vi "Puertas_Abiertas_3gdl.vi"() -> ()   [LabVIEW 2014]
uses:
  <vilib>/Platform/TimedLoop/XDataNode/timing_clust.ctl
  <vilib>/Platform/TimedLoop/XDataNode/nitl_modes.ctl
  <vilib>/Platform/TimedLoop/XDataNode/wakeup.ctl
  <vilib>/Analysis/baseanly.llb/Real A x B.vi
  <vilib>/Platform/TimedLoop/XDataNode/loadnilvce.vi
  <vilib>/Analysis/Matrix/Numeric/Conversions/Array To Matrix - RA2.vi
  <vilib>/Analysis/Matrix/Numeric/Conversions/Array To Matrix - RA.vi
  <vilib>/Motion/Express/_s/nimc.ex.read.readExecutionData.axis.vi
  Global_Inicial.vi
  <vilib>/platform/TimedLoop/XDataNode/XDataNode.xnode
  <vilib>/Motion/BlockNode/FB.NIMotion.xnode
  <vilib>/Platform/TimedLoop/XDataNode/XDNodeRunTimeDep.lvlib
  <vilib>/ptbypt/NI_PtbyPt.lvlib
  <vilib>/Analysis/NI_AALBase.lvlib
  <vilib>/Analysis/Matrix/NI_Matrix.lvlib
panel:
  in  "stop 2":bool
  in  "stop":bool
  out "pkt":bool
  out "Posición FEH":dbl
  out "Posición RotIEH":dbl
  out "Posición FEC":dbl
  out "error out":errorcluster
  out "position °":dbl
  out "inicial":dbl format="%#_13g"
  out "Pos ant":dbl
  out "V MOTOR abajo":dbl
  out "Pos ant 1":dbl
  out "qd - sin":dbl
  out "tau 1":dbl
  out "Time":u32
  out "Motor abajo":dynamicdata(graph)
  in  "Kp":dbl=40.0
  in  "M_p":dbl=14.0
  in  "Kd":dbl=40.0
  out "Error imp 1":dbl[](graph)
  out "inicial 2":dbl format="%#_13g"
  out "Pos ant 2":dbl
  out "position ° 2":dbl
  out "Pos ant 2_2":dbl
  out "Motor medio":dynamicdata(graph)
  out "Error imp 2":dbl[](graph)
  out "Motor superior":dynamicdata(graph)
  out "inicial 3":dbl format="%#_13g"
  out "Pos ant 3":dbl
  out "position ° 3":dbl
  out "Pos ant 3_3":dbl
  out "q1":dbl
  out "qhp1":dbl
  out "qhpp1":dbl
  out "qhpp2":dbl
  out "qhp2":dbl
  out "q2":dbl
  out "qhpp3":dbl
  out "qhp3":dbl
  out "q3":dbl
  out "V MOTOR medio":dbl
  out "tau 2":dbl
  out "V MOTOR  superior":dbl
  out "tau 3":dbl
  out "Trayectoria qd 1":dbl[](array[numeric])
  out "Trayectoria qd 2":dbl[](array[numeric])
  out "Trayectoria qd 3":dbl[](array[numeric])
  out "qe cal 2":dbl
  out "Error imp 3":dbl[](graph)
  in  "epsilon 2":dbl=0.001 format="%#_13g"
  in  "epsilon 1":dbl=0.001 format="%#_13g"
  in  "epsilon 3":dbl=0.01 format="%#_13g"
  in  "sat 1":dbl=2.0
  in  "sat 2":dbl=2.0
  in  "sat 3":dbl=2.0
  in  "sat 4":dbl=2.0
  in  "sat 5":dbl=2.0
  in  "sat 6":dbl=0.0001
  in  "sat 7":dbl=0.0001
  in  "sat 8":dbl=2.0
  in  "sat 9":dbl=2.0
  in  "sat 10":dbl=2.0
  in  "sat 11":dbl=2.0
  in  "sat 12":dbl=2.0
  in  "sat 13":dbl=2.0
  in  "sat 14":dbl=2.0
  in  "sat 15":dbl=2.0
  in  "sat 16":dbl=2.0
  in  "sat 17":dbl=0.001
  in  "sat 18":dbl=5.0
  in  "sat 19":dbl=2.0
  in  "sat 20":dbl=2.0
  in  "sat 21":dbl=2.0
  in  "g 1":dbl=10.0
  in  "g 2":dbl=10.0
  in  "g 3":dbl=10.0
  in  "g 4":dbl=10.0
  in  "g 5":dbl=10.0
  in  "g 6":dbl=0.01
  in  "g 7":dbl=0.01
  in  "g 8":dbl=10.0
  in  "g 9":dbl=10.0
  in  "g 10":dbl=10.0
  in  "g 11":dbl=10.0
  in  "g 12":dbl=10.0
  in  "g 13":dbl=10.0
  in  "g 14":dbl=10.0
  in  "g 15":dbl=10.0
  in  "g 16":dbl=10.0
  in  "g 17":dbl=10.0
  in  "g 18":dbl=10.0
  in  "g 19":dbl=10.0
  in  "g 20":dbl=10.0
  in  "g 21":dbl=10.0
  out "i":i32
  out "Y":dbl[][](array[numeric])
  out "Sp_kpE":dbl
  out "Sp_kpE 2":dbl
  out "Sp_kpE 3":dbl
  out "qe cal 1":dbl
  out "qe cal 3":dbl
  out "qd - sin 2":dbl
  in  "Kp 2":dbl=250.0
  in  "M_p 2":dbl=90.0
  in  "Kd 2":dbl=250.0
  out "qd - sin 3":dbl
  in  "Kp 3":dbl=100.0
  in  "M_p 3":dbl=20.0
  in  "Kd 3":dbl=100.0
  in  "timeout ms (25000)":i32=100
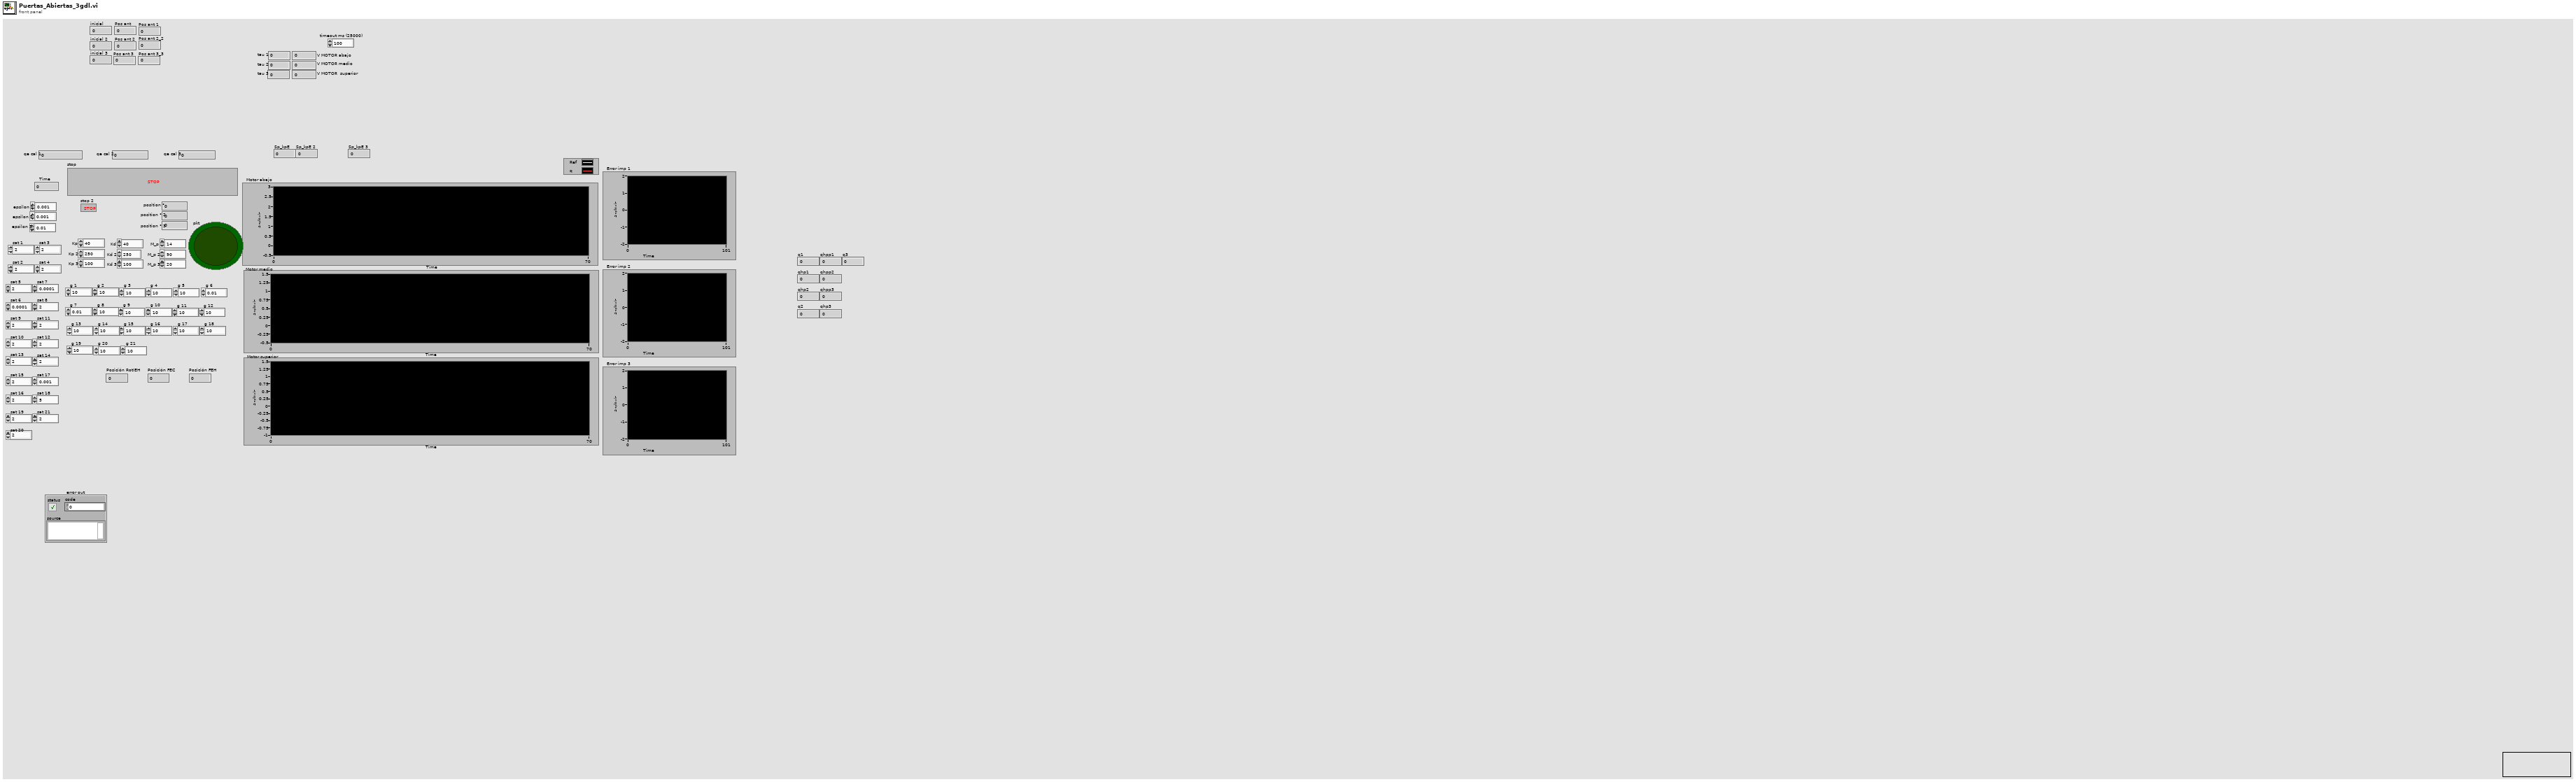
[diagram p1: front panel]
types:
  T1 = typedef "XDNodeRunTimeDep.lvlib/timing_clust.ctl" = cluster{"Expected End [f-1]":u64, "Actual End [f-1]":u64, "Finished Late? [f-1]":bool, "Expected End [i-1]":u64, "Actual End [i-1]":u64, "Finished Late? [i-1]":bool, "Expected Start [i]":u64, "Actual Start [i]":u64, "Expected Start [f]":u64, "Actual Start [f]":u64, "Source Name":string, "Structure Name":string, "Period":i64, "Deadline":i64, "Offset":i64, "Start":i64, "Priority":i32, "Timeout":i32, "Mode":T2, "Wakeup Reason":T3, "Error":errorcluster, "Source Type":string, "Secondary Source Type":string, "Global End Time":u64, "Global Start Time":u64, "Frame Duration":u64, "Iteration Duration":u64, "Assigned CPU":i32, "I/O Scan Engine Mode":u32}
  T2 = typedef "XDNodeRunTimeDep.lvlib/nitl_modes.ctl" = enum32{"No Change", "Process missed periods, maintain original phase", "Discard missed periods, maintain original phase", "Process missed periods, ignore original phase", "Discard missed periods, ignore original phase"}
  T3 = typedef "XDNodeRunTimeDep.lvlib/wakeup.ctl" = enum32{"Normal", "Aborted", "Asynchronous wakeup", "Timing source error", "Timed loop error", "Timeout"}
  T4 = typedef "NI_Matrix.lvlib/RealMatrix.ctl" = dbl[][]
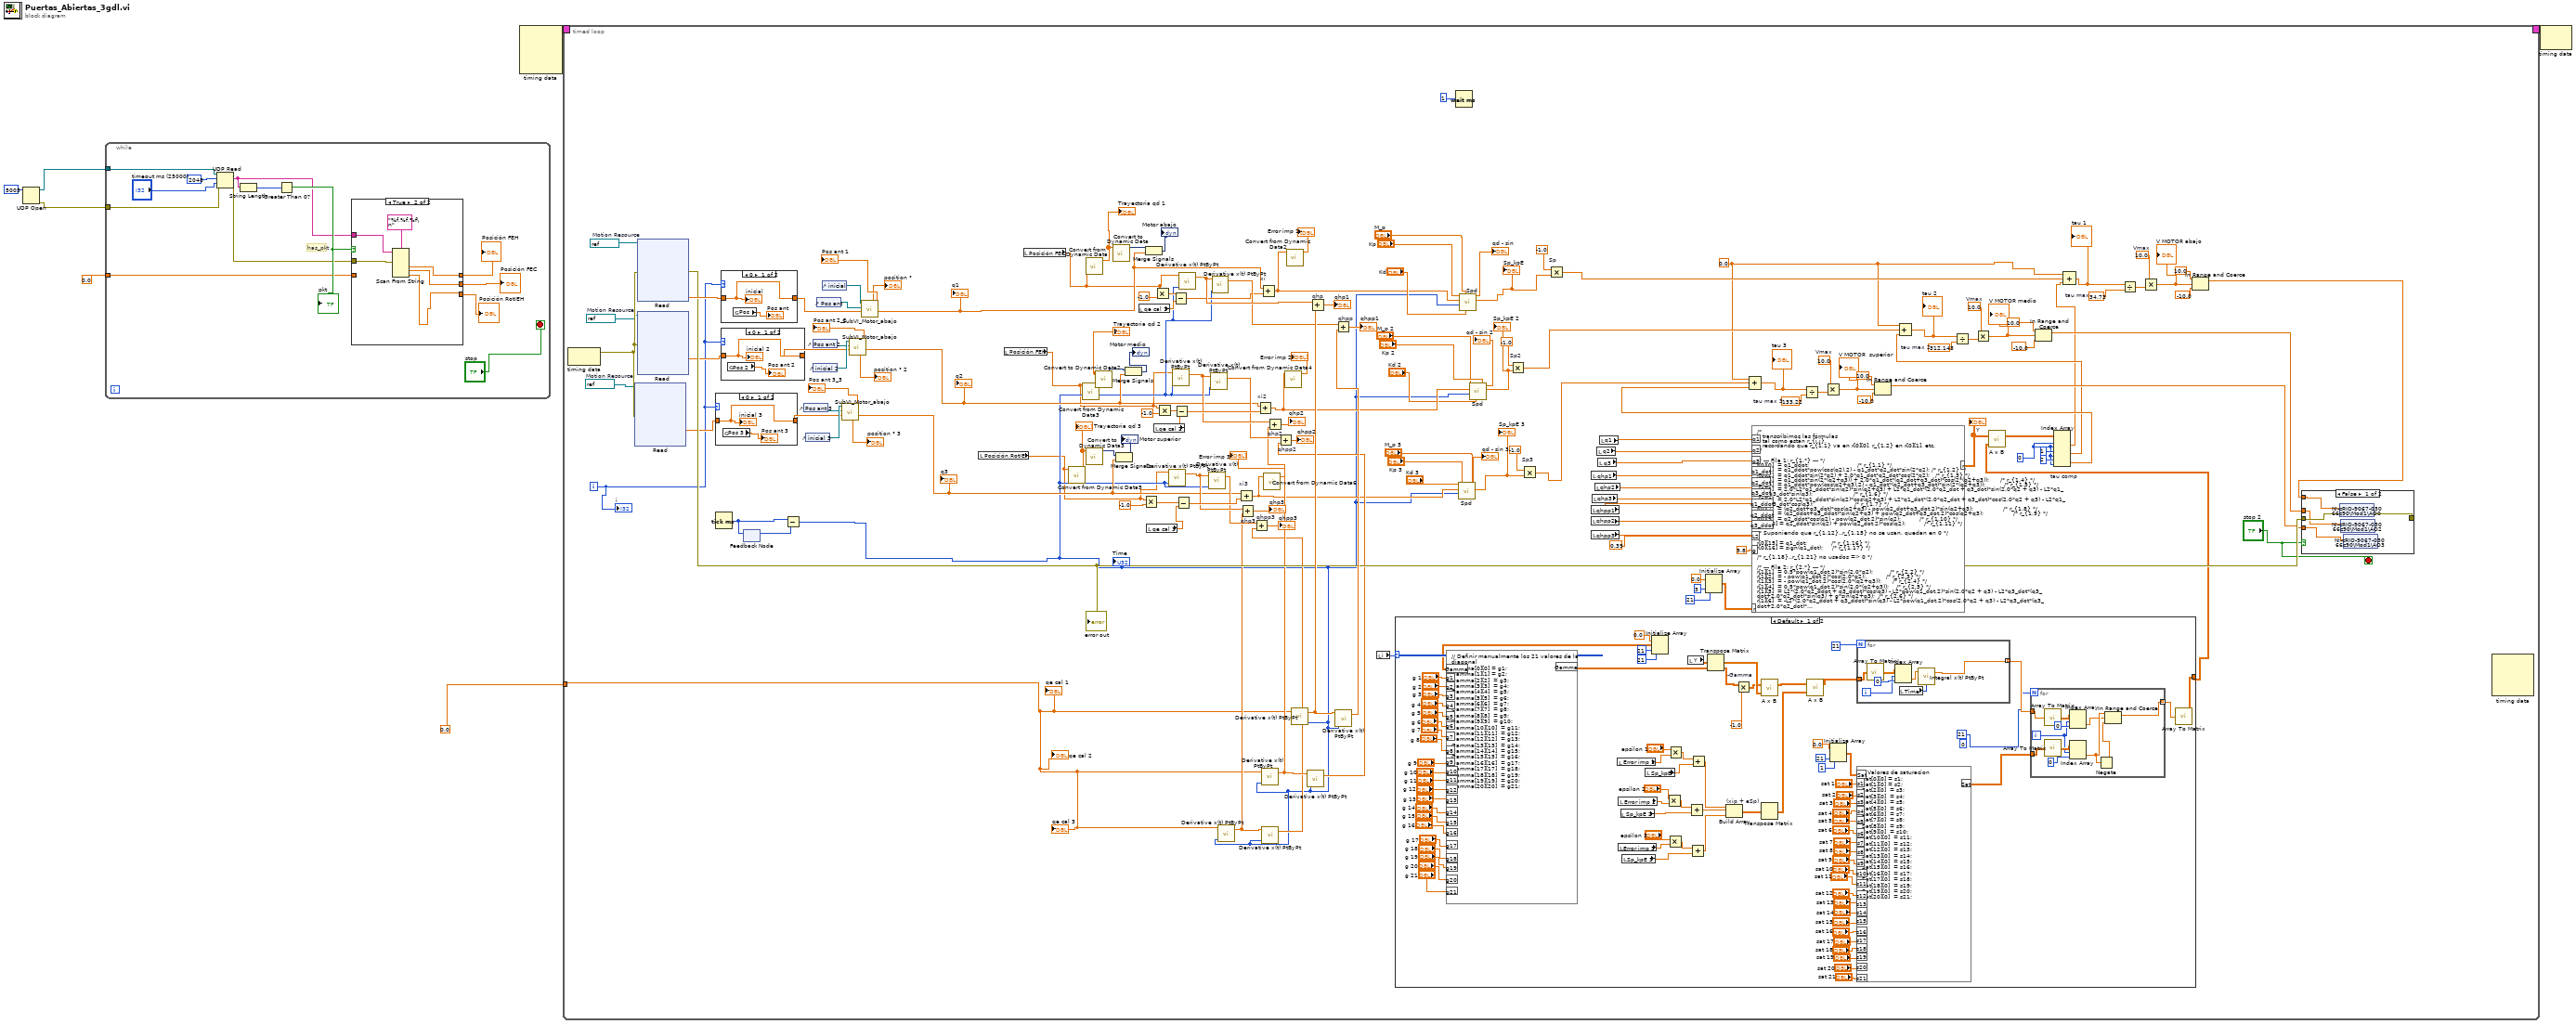
[diagram p0: block diagram]
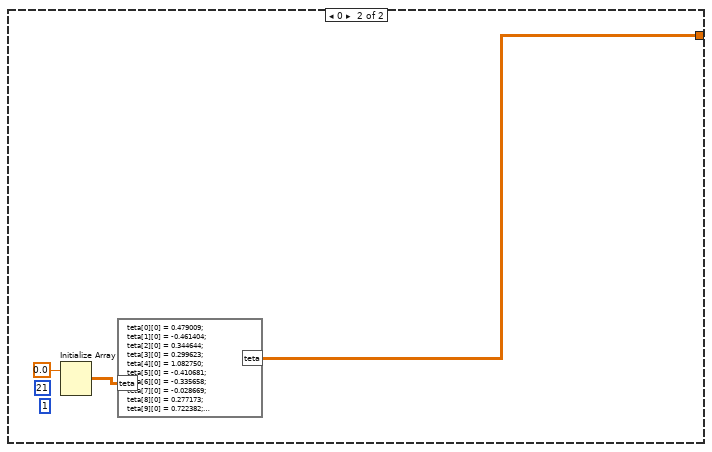
[diagram p2: hidden frame]
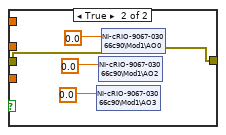
[diagram p5: hidden frame]
diagram:
  n1 = UDP Open(11:u16 5005 ("port")) -> (port=w6:refnum<k16>, 0:w7:errorcluster)  [unwired: 4 in, 1 out]
  n2 = while {
    tunnel: w7 -> [w17]
    tunnel: w6 -> [w16]
    tunnel: 0.0 -> [w11]
    stop <- "stop" stop-if-true
    # "has_pkt"
    n3 = UDP Read(connection ID=w16, max size (548)=2048, timeout ms (25000)="timeout ms (25000)", 8:w17) -> (data out=w13:string, error out=w12:errorcluster)  [unwired: 3 out]
    n4 = String Length(string=w13) -> (length=w18:i32)
    n5 = Greater Than 0?(x=w18) -> (x > 0?=w14:bool)
    "pkt" <- w14
    n6 = case shown="True" w14 {
      tunnel: w12 -> [_ w27]
      tunnel: w13 -> [_ w26]
      tunnel: [w21 w24] -> w15
      tunnel: w11 -> [w21 _]
      tunnel: [w21 w23] -> w10
      tunnel: [w21 w22] -> w9
      frame False {
      }
      frame True {
        n7 = Scan From String "Scan From String"(format string="%f,%f,%f\n", input string=w26, error in=w27) -> (output 1=w24:dbl, output 2=w23:dbl, output 3=w22:dbl)  [unwired: 4 in, 3 out]
      }
    }
    "Posición FEC" <- w10
    "Posición RotIEH" <- w9
    "Posición FEH" <- w15
  }
  n8 = node-c288() -> (w3:T1)  [unwired: 4 in]
  n9 = timed-loop {
    timing: w3 -> [_]
    timing-out: [_] -> w2
    tunnel: 0.0 -> [w33]
    i -> [w67]
    stop <- "stop 2" stop-if-true
    w32 = 0.0
    w70 = refnum<k21> "Axis 3"  # Motion Resource
    w71 = refnum<k21> "Axis 2"  # Motion Resource
    w88 = 0 ("index (col)")
    w95 = 10.0  # Vmax
    w97 = 133.22  # tau max 3
    w102 = 10.0  # Vmax
    w104 = 312.143  # tau max 2
    w177 = 10.0  # Vmax
    w179 = 34.73  # tau max
    w157 = refnum<k21> "Axis 1"  # Motion Resource
    n10 = node-c288() -> (w152:errorcluster)  [unwired: 1 in]
    n11 = xnode ("Read")("resource"=w71, "error in"=w152) -> ("position"=w121:dbl)  [unwired: 6 out]
    n12 = xnode ("Read")("resource"=w157, "error in"=w152) -> ("position"=w176:dbl, "error out"=w166:errorcluster)  [unwired: 5 out]
    "error out" <- w166
    n13 = xnode ("Read")("resource"=w70, "error in"=w152) -> ("position"=w151:dbl)  [unwired: 6 out]
    n14 = case shown="0" w67 {
      tunnel: w121 -> [w282 w283]
      tunnel: [w282 w283] -> w122
      frame 0 {
        n15 = global read "Global_Inicial.vi" "Pos 3"() -> (→"Pos ant 3":dbl)
        "inicial 3" <- w282
      }
      frame Default {
      }
    }
    n16 = Tick Count (ms)() -> (millisecond timer value=w68:u32)
    n17 = case shown="0" w67 {
      tunnel: w176 -> [w316 w317]
      tunnel: [w316 w317] -> w175
      frame 0 {
        n18 = global read "Global_Inicial.vi" "Pos"() -> (→"Pos ant":dbl)
        "inicial" <- w316
      }
      frame Default {
      }
    }
    n19 = case shown="0" w67 {
      tunnel: w151 -> [w285 w286]
      tunnel: [w285 w286] -> w146
      frame 0 {
        n20 = global read "Global_Inicial.vi" "Pos 2"() -> (→"Pos ant 2":dbl)
        "inicial 2" <- w285
      }
      frame Default {
      }
    }
    n21 = feedback #1() -> (w69:u32)  [unwired: 1 in]
    n22 = feedback-in #1(w68) -> ()
    n23 = Subtract(x=w68, y=w69) -> (x-y=w37:u32)
    "Time" <- w37
    n24 = control-ref of="Pos ant 3"() -> (w125:refnum<vi>)
    n25 = control-ref of="inicial 3"() -> (w126:refnum<vi>)
    n26 = control-ref of="Pos ant 2"() -> (w149:refnum<vi>)
    n27 = control-ref of="inicial 2"() -> (w150:refnum<vi>)
    n28 = control-ref of="Pos ant"() -> (w155:refnum<vi>)
    n29 = control-ref of="inicial"() -> (w156:refnum<vi>)
    n30 = call "SubVI_Motor_abajo.vi"("position"=w122, "reference in"=w125, "Digital in"=w126) -> ("Numeric"=w77:dbl, "Pos ant 2"=→"Pos ant 3_3":dbl, "position °"=→"position ° 3":dbl)  [unwired: 5 in, 1 out]
    "q3" <- w77
    n31 = call "SubVI_Motor_abajo.vi"("position"=w146, "reference in"=w149, "Digital in"=w150) -> ("Numeric"=w59:dbl, "Pos ant 2"=→"Pos ant 2_2":dbl, "position °"=→"position ° 2":dbl)  [unwired: 5 in, 1 out]
    "q2" <- w59
    n32 = call "SubVI_Motor_abajo.vi"("position"=w175, "reference in"=w155, "Digital in"=w156) -> ("Numeric"=w140:dbl, "Pos ant 2"=→"Pos ant 1":dbl, "position °"=→"position °":dbl)  [unwired: 5 in, 1 out]
    "q1" <- w140
    n33 = local read "Posición RotIEH"() -> (w29:dbl)
    n34 = local read "Posición FEH"() -> (w31:dbl)
    n35 = local read "Posición FEC"() -> (w30:dbl)
    n36 = call "Convert from Dynamic Data5"("Dynamic Data Type"=w29) -> ("Array"=w79:dbl[])  [unwired: 3 in]
    "Trayectoria qd 3" <- w79
    n37 = call "Convert from Dynamic Data3"("Dynamic Data Type"=w31) -> ("Array"=w80:dbl[])  [unwired: 3 in]
    "Trayectoria qd 2" <- w80
    n38 = call "Convert from Dynamic Data"("Dynamic Data Type"=w30) -> ("Array"=w145:dbl[])  [unwired: 3 in]
    "Trayectoria qd 1" <- w145
    n39 = call "Convert to Dynamic Data3"("Array"=w79) -> ("Dynamic Data Type"=w135:dynamicdata)  [unwired: 3 in]
    n40 = call "Convert to Dynamic Data2"("Array"=w80) -> ("Dynamic Data Type"=w78:dynamicdata)  [unwired: 3 in]
    n41 = call "Convert to Dynamic Data"("Array"=w145) -> ("Dynamic Data Type"=w164:dynamicdata)  [unwired: 3 in]
    n42 = Merge Signals(w135, w77) -> (→"Motor superior":dynamicdata)
    n43 = Merge Signals(w78, w59) -> (→"Motor medio":dynamicdata)
    n44 = local read "qe cal 1"() -> (w58:dbl)
    n45 = Multiply(x=w29, y=-1.0) -> (x*y=w132:dbl)
    n46 = Merge Signals(w164, w140) -> (→"Motor abajo":dynamicdata)
    n47 = local read "qe cal 3"() -> (w56:dbl)
    n48 = local read "qe cal 2"() -> (w57:dbl)
    n49 = Multiply(x=w30, y=-1.0) -> (x*y=w162:dbl)
    n50 = Multiply(x=w31, y=-1.0) -> (x*y=w143:dbl)
    n51 = call <vilib>:"Derivative x(t) PtByPt.vi"("dt"=w37, "x"=w29) -> ("dx/dt"=w130:dbl)  [unwired: 2 in, 1 out]
    n52 = Subtract(x=w162, y=w58) -> (x-y=w161:dbl)
    n53 = call <vilib>:"Derivative x(t) PtByPt.vi"("dt"=w37, "x"=w31) -> ("dx/dt"=w138:dbl)  [unwired: 2 in, 1 out]
    n54 = Subtract(x=w143, y=w57) -> (x-y=w141:dbl)
    n55 = Subtract(x=w132, y=w56) -> (x-y=w131:dbl)
    n56 = call <vilib>:"Derivative x(t) PtByPt.vi"("dt"=w37, "x"=w30) -> ("dx/dt"=w170:dbl)  [unwired: 2 in, 1 out]
    n57 = call <vilib>:"Derivative x(t) PtByPt.vi"("dt"=w37, "x"=w130) -> ("dx/dt"=w129:dbl)  [unwired: 2 in, 1 out]
    n58 = call <vilib>:"Derivative x(t) PtByPt.vi"("dt"=w37, "x"=w138) -> ("dx/dt"=w137:dbl)  [unwired: 2 in, 1 out]
    n59 = call <vilib>:"Derivative x(t) PtByPt.vi"("dt"=w37, "x"=w170) -> ("dx/dt"=w168:dbl)  [unwired: 2 in, 1 out]
    n60 = call <vilib>:"Derivative x(t) PtByPt.vi"("dt"=w37, "x"=w33) -> ("dx/dt"=w82:dbl)  [unwired: 2 in, 1 out]
    n61 = Add "xi3"(x=w77, y=w131) -> (x+y=w38:dbl)
    n62 = Add "qhp3"(x=w130, y=w82) -> (x+y=→"qhp3":dbl)
    n63 = Add "xi2"(x=w59, y=w141) -> (x+y=w45:dbl)
    n64 = Add "xi"(x=w140, y=w161) -> (x+y=w51:dbl)
    n65 = call <vilib>:"Derivative x(t) PtByPt.vi"("dt"=w37, "x"=w33) -> ("dx/dt"=w84:dbl)  [unwired: 2 in, 1 out]
    n66 = call <vilib>:"Derivative x(t) PtByPt.vi"("dt"=w37, "x"=w82) -> ("dx/dt"=w81:dbl)  [unwired: 2 in, 1 out]
    n67 = Add "qhpp3"(x=w129, y=w81) -> (x+y=→"qhpp3":dbl)
    n68 = call "Convert from Dynamic Data6"("Dynamic Data Type"=w38) -> ("Array"=→"Error imp 3":dbl[])  [unwired: 3 in]
    n69 = Add "qhp2"(x=w138, y=w84) -> (x+y=→"qhp2":dbl)
    n70 = call "Convert from Dynamic Data4"("Dynamic Data Type"=w45) -> ("Array"=→"Error imp 2":dbl[])  [unwired: 3 in]
    n71 = call "Convert from Dynamic Data2"("Dynamic Data Type"=w51) -> ("Array"=→"Error imp 1":dbl[])  [unwired: 3 in]
    n72 = call <vilib>:"Derivative x(t) PtByPt.vi"("dt"=w37, "x"=w33) -> ("dx/dt"=w169:dbl)  [unwired: 2 in, 1 out]
    n73 = call <vilib>:"Derivative x(t) PtByPt.vi"("dt"=w37, "x"=w84) -> ("dx/dt"=w83:dbl)  [unwired: 2 in, 1 out]
    n74 = Add "qhpp2"(x=w137, y=w83) -> (x+y=→"qhpp2":dbl)
    n75 = Add "qhp"(x=w170, y=w169) -> (x+y=→"qhp1":dbl)
    n76 = call <vilib>:"Derivative x(t) PtByPt.vi"("dt"=w37, "x"=w169) -> ("dx/dt"=w167:dbl)  [unwired: 2 in, 1 out]
    n77 = Add "qhpp"(x=w168, y=w167) -> (x+y=→"qhpp1":dbl)
    n78 = local read "i"() -> (w66:i32)
    n79 = case shown="Default" w66 {
      tunnel: [w224 w278] -> w60
      frame Default {
        (unwired) 0 ("dimension size")
        n80 = local read "Error imp 1"() -> (w249:dbl[])
        n81 = local read "Error imp 3"() -> (w240:dbl[])
        n82 = local read "Error imp 2"() -> (w244:dbl[])
        n83 = local read "Sp_kpE 2"() -> (w243:dbl)
        n84 = local read "Sp_kpE 3"() -> (w239:dbl)
        n85 = local read "Sp_kpE"() -> (w247:dbl)
        n86 = Initialize Array(0.0 ("element"), 21 ("dimension size"), 21 ("dimension size")) -> (w255:dbl[][])
        n87 = formula code="// Definir manualmente los 21 valores de la diagonal\nGamma[0][0] = g1;\nGamma[1][1] = g2;\nGamma[2][2]  = g3;\nGamma[3][3]  = g4;\nGamma[4][4]  = g5;\nGamma[5][5]  = g6;\nGamma[6][6]  = g7;\nGamma[7][7]  = g8;\nGamma[8][8]  = g9;\nGamma[9][9]  = g10;\nGamma[10][10]  = g11;\nGamma[11][11]  = g12;\nGamma[12][12]  = g13;\nGamma[13][13]  = g14;\nGamma[14][14]  = g15;\nGamma[15][15]  = g16;\nGamma[16][16]  = g17;\nGamma[17][17]  = g18;\nGamma[18][18]  = g19;\nGamma[19][19]  = g20;\nGamma[20][20]  = g21;"("Gamma"=w255, "g1"="g 1", "g2"="g 2", "g3"="g 3", "g4"="g 4", "g5"="g 5", "g6"="g 6", "g7"="g 7", "g8"="g 8", "g9"="g 9", "g10"="g 10", "g11"="g 11", "g12"="g 12", "g13"="g 13", "g14"="g 14", "g15"="g 15", "g16"="g 16", "g17"="g 17", "g18"="g 18", "g19"="g 19", "g20"="g 20", "g21"="g 21") -> ("Gamma"=w253:dbl[][])
        n88 = Multiply(x="epsilon 2", y=w244) -> (x*y=w246:dbl[])
        n89 = Multiply(x="epsilon 3", y=w240) -> (x*y=w242:dbl[])
        n90 = Multiply(x="epsilon 1", y=w249) -> (x*y=w248:dbl[])
        n91 = local read "Y"() -> (w259:dbl[][])
        n92 = Add(x=w246, y=w243) -> (x+y=w237:dbl[])
        n93 = Add(x=w242, y=w239) -> (x+y=w236:dbl[])
        n94 = Add(x=w248, y=w247) -> (x+y=w238:dbl[])
        n95 = Transpose Matrix(1:w259) -> (0:w254:dbl[][])
        n96 = Build Array "(xip + eSp)"(w238, w237, w236) -> (w228:T4)
        n97 = Multiply "-Gamma"(x=w253, y=-1.0) -> (x*y=w252:dbl[][])
        n98 = Transpose Matrix(1:w228) -> (0:w227:T4)
        n99 = call-poly <vilib>:"A x B.vi"("B"=w254, "A"=w252) -> ("A x B"=w251:T4)  [unwired: 1 out]
        n100 = call-poly <vilib>:"A x B.vi"("B"=w227, "A"=w251) -> ("A x B"=w235:T4)  [unwired: 1 out]
        n101 = Initialize Array(0.0 ("element"), 21 ("dimension size"), 1 ("dimension size")) -> (w231:dbl[][])
        n102 = for {
          N: 21 ("dimension size") -> [_]
          tunnel: w235 -> [w273]
          tunnel: [w271] -> w226 mode=indexing
          i -> [w275]
          n103 = call-poly <vilib>:"Array To Matrix.vi"("Real 2D Array"=w273) -> ("Real Matrix"=w274:T4)
          n104 = Index Array(array=w274, index (row)=w275, index (col)=0) -> (element=w272:dbl)
          n105 = local read "Time"() -> (w276:u32)
          n106 = call <vilib>:"Integral x(t) PtByPt.vi"("dt"=w276, "x"=w272) -> ("integral x(t)"=w271:dbl)  [unwired: 2 in, 1 out]
        }
        n107 = formula code="// Valores de saturacion\nSat[0][0] = s1;\nSat[1][0] = s2;\nSat[2][0]  = s3;\nSat[3][0]  = s4;\nSat[4][0]  = s5;\nSat[5][0]  = s6;\nSat[6][0]  = s7;\nSat[7][0]  = s8;\nSat[8][0]  = s9;\nSat[9][0]  = s10;\nSat[10][0]  = s11;\nSat[11][0]  = s12;\nSat[12][0]  = s13;\nSat[13][0]  = s14;\nSat[14][0]  = s15;\nSat[15][0]  = s16;\nSat[16][0]  = s17;\nSat[17][0]  = s18;\nSat[18][0]  = s19;\nSat[19][0]  = s20;\nSat[20][0]  = s21;"("Sat"=w231, "s1"="sat 1", "s2"="sat 2", "s3"="sat 3", "s4"="sat 4", "s5"="sat 5", "s6"="sat 6", "s7"="sat 7", "s8"="sat 8", "s9"="sat 9", "s10"="sat 10", "s11"="sat 11", "s12"="sat 12", "s13"="sat 13", "s14"="sat 14", "s15"="sat 15", "s16"="sat 16", "s17"="sat 17", "s18"="sat 18", "s19"="sat 19", "s20"="sat 20", "s21"="sat 21") -> ("Sat"=w230:dbl[][])
        n108 = for {
          N: 21 ("dimension size") -> [_]
          tunnel: w226 -> [w270]
          tunnel: w230 -> [w266]
          tunnel: [w260] -> w225 mode=indexing
          i -> [w261]
          n109 = call-poly <vilib>:"Array To Matrix.vi"("Real 2D Array"=w266) -> ("Real Matrix"=w267:T4)
          n110 = call-poly <vilib>:"Array To Matrix.vi"("Real 1D Array"=w270) -> ("Real Matrix (Column Vector)"=w269:T4)
          n111 = Index Array(array=w267, index (row)=w261, index (col)=0) -> (element=w264:dbl)
          n112 = Index Array(array=w269, index (row)=w261, index (col)=0) -> (element=w262:dbl)
          n113 = Negate(x=w264) -> (-x=w263:dbl)
          n114 = In Range and Coerce(upper limit=w264, x=w262, lower limit=w263) -> (coerced(x)=w260:dbl)  [unwired: 1 out]
        }
        n115 = call-poly <vilib>:"Array To Matrix.vi"("Real 1D Array"=w225) -> ("Real Matrix (Column Vector)"=w224:T4)
      }
      frame 0 {
        (unwired) 1 ("dimension size")
        (unwired) 21 ("dimension size")
        n116 = Initialize Array(0.0 ("element")) -> (w279:dbl[][])  [unwired: 2 in]
        n117 = formula code="teta[0][0] = 0.479009;\nteta[1][0] = -0.461404;\nteta[2][0] = 0.344644;\nteta[3][0] = 0.299623;\nteta[4][0] = 1.082750;\nteta[5][0] = -0.410681;\nteta[6][0] = -0.335658;\nteta[7][0] = -0.028669;\nteta[8][0] = 0.277173;\nteta[9][0] = 0.722382;\nteta[10][0] = 0.110651;\nteta[11][0] = 1.224468;\nteta[12][0] = -0.093521;\nteta[13][0] = 9.464194;\nteta[14][0] = -0.583702;\nteta[15][0] = 7.453121;\nteta[16][0] = 6.357999;\nteta[17][0] = 4.094850;\nteta[18][0] = 6.671452;\nteta[19][0] = 0.063043;\nteta[20][0] = -0.211661;"("teta"=w279) -> ("teta"=w278:dbl[][])
      }
    }
    n118 = Wait (ms)(milliseconds to wait=u32 1) -> ()  [unwired: 1 out]
    n119 = call "Spd.vi"("Kd in"="Kd 3", "M_p in"="M_p 3", "Numeric"=w37, "Dynamic Data"=w38, "Kp in"="Kp 3") -> ("Spd"=w39:dbl, "qd - sin 4"=→"qd - sin 3":dbl)  [unwired: 5 in]
    "Sp_kpE 3" <- w39
    n120 = call "Spd.vi"("Kd in"="Kd", "M_p in"="M_p", "Numeric"=w37, "Dynamic Data"=w51, "Kp in"="Kp") -> ("Spd"=w50:dbl, "qd - sin 4"=→"qd - sin":dbl)  [unwired: 5 in]
    "Sp_kpE" <- w50
    n121 = call "Spd.vi"("Kd in"="Kd 2", "M_p in"="M_p 2", "Numeric"=w37, "Dynamic Data"=w45, "Kp in"="Kp 2") -> ("Spd"=w46:dbl, "qd - sin 4"=→"qd - sin 2":dbl)  [unwired: 5 in]
    "Sp_kpE 2" <- w46
    n122 = Multiply "Sp2"(x=-1.0, y=w46) -> (x*y=w48:dbl)
    n123 = Multiply "Sp3"(x=-1.0, y=w39) -> (x*y=w41:dbl)
    n124 = Multiply "Sp"(x=-1.0, y=w50) -> (x*y=w49:dbl)
    n125 = local read "qhpp1"() -> (w115:dbl)
    n126 = local read "qhpp2"() -> (w112:dbl)
    n127 = local read "qhpp3"() -> (w107:dbl)
    n128 = local read "qhp1"() -> (w116:dbl)
    n129 = local read "qhp3"() -> (w106:dbl)
    n130 = local read "qhp2"() -> (w111:dbl)
    n131 = local read "q2"() -> (w110:dbl)
    n132 = local read "q3"() -> (w105:dbl)
    n133 = local read "q1"() -> (w117:dbl)
    n134 = Initialize Array(0.0 ("element"), 3 ("dimension size"), 21 ("dimension size")) -> (w65:dbl[][])
    n135 = formula code="/* \n   transcribimos las fórmulas \n   tal como están r_{i,j}, \n   recordando que r_{1,1} va en r[0][0], r_{1,2} en r[0][1], etc.\n*/\n\n/* --- Fila 1: r_{1,*} --- */\nr[0][0]  = q1_ddot;                          /* r_{1,1} */\nr[0][1]  = q1_ddot*pow(cos(q2),2) - q1_dot*q2_dot*sin(2*q2); /* r_{1,2} */\nr[0][2]  = q1_ddot*sin(2*q2) + 2.0*q1_dot*q2_dot*cos(2*q2);   /* r_{1,3} */\nr[0][3]  = q1_ddot*sin(2*(q2+q3)) + 2.0*q1_dot*(q2_dot+q3_dot)*cos(2*(q2+q3));      /* r_{1,4} */\nr[0][4]  = q1_ddot*pow(cos(q2+q3),2) - q1_dot*(q2_dot+q3_dot)*sin(2*(q2+q3));          /* r_{1,5} */\nr[0][5]  = 2.0*L2*q1_ddot*sin(q2)*sin(q2+q3) + L2*q1_dot*(2.0*q2_dot + q3_dot)*sin(2.0*q2 + q3) - L2*q1_dot*q3_dot*sin(q3);                      /* r_{1,6} */\nr[0][6]  = 2.0*L2*q1_ddot*sin(q2)*cos(q2+q3) + L2*q1_dot*(2.0*q2_dot + q3_dot)*cos(2.0*q2 + q3) - L2*q1_dot*q3_dot*cos(q3);                      /* r_{1,7} */\nr[0][7]  = (q2_dot+q3_dot)*cos(q2+q3) - pow(q2_dot+q3_dot,2)*sin(q2+q3);                /* r_{1,8} */\nr[0][8]  = (q2_ddot+q3_ddot)*sin(q2+q3) + pow(q2_dot+q3_dot,2)*cos(q2+q3);                /* r_{1,9} */\nr[0][9]  = q2_ddot*cos(q2) - pow(q2_dot,2)*sin(q2);          /* r_{1,10} */\nr[0][10] = q2_ddot*sin(q2) + pow(q2_dot,2)*cos(q2);          /* r_{1,11} */\n\n/* Suponiendo que r_{1,12}..r_{1,15} no se usan, quedan en 0 */\n\nr[0][15] = q1_dot;             /* r_{1,16} */\nr[0][16] = sign(q1_dot);     /* r_{1,17} */\n\n/* r_{1,18}..r_{1,21} no usados => 0 */\n\n/* --- Fila 2: r_{2,*} --- */\nr[1][1]  = 0.5*pow(q1_dot,2)*sin(2.0*q2);         /* r_{2,2} */\nr[1][2]  = - pow(q1_dot,2)*cos(2.0*q2);           /* r_{2,3} */\nr[1][3]  = - pow(q1_dot,2)*cos(2.0*(q2+q3));      /* r_{2,4} */\nr[1][4]  = 0.5*pow(q1_dot,2)*sin(2.0*(q2+q3));    /* r_{2,5} */\nr[1][5]  = L2*(2.0*q2_ddot + q3_ddot)*cos(q3) - L2*pow(q1_dot,2)*sin(2.0*q2 + q3) - L2*q3_dot*(q3_dot+2.0*q2_dot)*sin(q3) + g*sin(q2+q3);  /* r_{2,6} */\nr[1][6]  = -L2*(2.0*q2_ddot + q3_ddot)*sin(q3) - L2*pow(q1_dot,2)*cos(2.0*q2 + q3) - L2*q3_dot*(q3_dot+2.0*q2_dot)*cos(q3) + g*cos(q2+q3);  /* r_{2,7} */\nr[1][7]  = q1_ddot*cos(q2+q3);    /* r_{2,8} */\nr[1][8]  = q1_ddot*sin(q2+q3);    /* r_{2,9} */\nr[1][9]  = q1_ddot*cos(q2);       /* r_{2,10} */\nr[1][10] = q1_ddot*sin(q2);       /* r_{2,11} */\nr[1][11] = q2_ddot;              /* r_{2,12} */\nr[1][12] = q3_ddot;              /* r_{2,13} */\nr[1][13] = sin(q2);              /* r_{2,14} */\nr[1][14] = cos(q2);              /* r_{2,15} */\n/* r_{2,16}, r_{2,17} => 0 */\nr[1][17] = q2_dot;               /* r_{2,18} */\nr[1][18] = sign(q2_dot);       /* r_{2,19} */\n/* r_{2,20}, r_{2,21} => 0 */\n\n/* --- Fila 3: r_{3,*} --- */\n/* r_{3,4}, r_{3,5}, r_{3,6}, r_{3,7}, r_{3,8}, r_{3,9}, etc. */\n\nr[2][3] = - pow(q1_dot,2)*cos(2.0*(q2+q3));   /* r_{3,4} */\nr[2][4] = 0.5*pow(q1_dot,2)*sin(2.0*(q2+q3)); /* r_{3,5} */\n\nr[2][5] = L2*q2_ddot*cos(q3) + 0.5*L2*pow(q1_dot,2)*( sin(q3) - sin(2.0*q2 + q3 ) ) + L2*pow(q2_dot,2)*sin(q3) + g*sin(q2+q3);        /* r_{3,6}, */\nr[2][6] = -L2*q2_ddot*sin(q3)  + 0.5*L2*pow(q1_dot,2)*( cos(q3) - cos(2.0*q2 + q3) )+ L2*pow(q2_dot,2)*cos(q3) + g*cos(q2+q3);        /* r_{3,7},  */\n\nr[2][7] = q1_ddot*cos(q2+q3);    /* r_{3,8} */\nr[2][8] = q1_ddot*sin(q2+q3);    /* r_{3,9} */\n\n/* r_{3,13} = q2_ddot + q3_ddot */\nr[2][12] = q2_ddot + q3_ddot;   /* r_{3,13} */\n\n/* r_{3,20} = q3_dot; r_{3,21} = sgn(q3_dot) */\nr[2][19] = q3_dot;              /* r_{3,20} */\nr[2][20] = sign(q3_dot);      /* r_{3,21} */"("q1"=w117, "q2"=w110, "q3"=w105, "q1_dot"=w116, "q2_dot"=w111, "q3_dot"=w106, "q1_ddot"=w115, "q2_ddot"=w112, "q3_ddot"=w107, "L2"=0.39 ("input variable"), "r"=w65, "g"=9.8 ("input variable")) -> ("r"=w127:dbl[][])
    "Y" <- w127
    n136 = call-poly <vilib>:"A x B.vi"("B"=w60, "A"=w127) -> ("A x B"=w87:T4)  [unwired: 1 out]
    n137 = Index Array "tau comp"(array=w87, index (row) #1=w88, index (col) #1=w88, index (row) #2=1 ("index (row)"), index (col) #2=w88, index (row) #3=2 ("index (row)"), index (col) #3=w88) -> (element #1=w62:dbl, element #2=w63:dbl, element #3=w64:dbl)
    n138 = Compound Arithmetic op=ADD(w32, w41, w64) -> (w91:dbl)
    "tau 3" <- w91
    n139 = Divide(x=w91, y=w97) -> (x/y=w96:dbl)
    n140 = Multiply ("Multiply.vi")(x=w95, y=w96) -> (x*y=w92:dbl)
    "V MOTOR  superior" <- w92
    n141 = In Range and Coerce(upper limit=10.0, x=w92, lower limit=-10.0) -> (coerced(x)=w85:dbl)  [unwired: 1 out]
    n142 = Compound Arithmetic op=ADD(w32, w48, w63) -> (w98:dbl)
    "tau 2" <- w98
    n143 = Divide(x=w98, y=w104) -> (x/y=w103:dbl)
    n144 = Multiply ("Multiply.vi")(x=w102, y=w103) -> (x*y=w99:dbl)
    "V MOTOR medio" <- w99
    n145 = In Range and Coerce(upper limit=10.0, x=w99, lower limit=-10.0) -> (coerced(x)=w86:dbl)  [unwired: 1 out]
    n146 = Compound Arithmetic op=ADD(w32, w49, w62) -> (w160:dbl)
    "tau 1" <- w160
    n147 = Divide(x=w160, y=w179) -> (x/y=w178:dbl)
    n148 = Multiply ("Multiply.vi")(x=w177, y=w178) -> (x*y=w172:dbl)
    "V MOTOR abajo" <- w172
    n149 = In Range and Coerce(upper limit=10.0, x=w172, lower limit=-10.0) -> (coerced(x)=w73:dbl)  [unwired: 1 out]
    n150 = case shown="False" "stop 2" {
      tunnel: w166 -> [w309 w313]
      tunnel: w73 -> [w308 _]
      tunnel: [w307 w312] -> _
      tunnel: w86 -> [w306 _]
      tunnel: w85 -> [w305 _]
      frame False {
        n151 = shared-variable "NI-cRIO-9067-03066c90\\Mod1\\AO0"(w308, error in=w309) -> (error out=w307:errorcluster)
        n152 = shared-variable "NI-cRIO-9067-03066c90\\Mod1\\AO2"(w306) -> ()  [unwired: 1 in, 1 out]
        n153 = shared-variable "NI-cRIO-9067-03066c90\\Mod1\\AO3"(w305) -> ()  [unwired: 1 in, 1 out]
      }
      frame True {
        n154 = shared-variable "NI-cRIO-9067-03066c90\\Mod1\\AO3"(0.0) -> ()  [unwired: 1 in, 1 out]
        n155 = shared-variable "NI-cRIO-9067-03066c90\\Mod1\\AO2"(0.0) -> ()  [unwired: 1 in, 1 out]
        n156 = shared-variable "NI-cRIO-9067-03066c90\\Mod1\\AO0"(0.0, error in=w313) -> (error out=w312:errorcluster)
      }
    }
    n157 = node-c288() -> ()  [unwired: 4 in, 1 out]
    "qe cal 2" <- w33
    "i" <- w67
    "qe cal 1" <- w33
    "qe cal 3" <- w33
  }
  n158 = node-c288(w2) -> ()  [unwired: 1 out]
